vi "Behaviors and stuff in progress.vi"() -> ()   [LabVIEW 2016]
uses:
  <vilib>/platform/TimedLoop/XDataNode/XDataNode.xnode
  <vilib>/Platform/TimedLoop/XDataNode/nitl_modes.ctl
  <vilib>/Platform/TimedLoop/XDataNode/XDNodeRunTimeDep.lvlib
  <vilib>/Platform/TimedLoop/XDataNode/wakeup.ctl
  <vilib>/Platform/TimedLoop/XDataNode/timing_clust.ctl
  Intake Commands.ctl
  <vilib>/Rock Robotics/SystemInterfaces/DIO/FPGA_DIOPWMChannel.ctl
  <vilib>/Rock Robotics/WPI/PWM/WPI_PWMDeadband.ctl
  <vilib>/Rock Robotics/WPI/MotorControl/WPI_MotorControlType.ctl
  <vilib>/Rock Robotics/WPI/MotorControl/WPI_MotorControlDeviceRef.ctl
panel:
  in  "Softstop":dbl
  in  "bottomInvert":bool
  in  "topInvert":bool
  in  "RpmThreshold":dbl
  in  "RpmStableVal":dbl
  in  "?":T1
  in  "MotorControlDevRef 2":T2={"DeviceStatus"={"status"=FALSE, "code"=0, "source"=""}, "Type"=enum."PWM", "PWM"={"PWM Channel"=enum."Invalid", "DeadBand"={"Name"="", "maxPositivePwm"=0, "minPositivePwm"=0, "centerPwm"=0, "maxNegativePwm"=0, "minNegativePwm"=0, "angularRange"=0}}, "CAN"={"Device Number"=0, "SetOutput VI Ref"=variant(enum8{"Percent VBus", "Current", "Speed", "Position", "Voltage"} enum."Percent VBus"), "GetOutput VI Ref"=variant(refnum<k1> refnum), "Enable VI Ref"=variant(dbl 12.0), "Disable VI Ref"=variant(enum8{"Percent VBus", "Speed", "Position", "Slave", "Unchanged / Invalid"} enum."Percent VBus"), "Data"=variant}, "Invert"=FALSE}
  in  "Carousel Invert?":bool
  in  "Conveyor Invert?":bool
  in  "bottomPIDF":T6
  in  "topPIDF":T7
  in  "Desired Angle 2":dbl
  in  "Desired Angle":dbl
  in  "Carousel motorInput":dbl
  in  "Conveyor motorInput":dbl
  in  "output range":cluster{"output high":dbl, "output low":dbl}={"output high"=1.0, "output low"=-1.0}
  in  "PID gains":T8={"proportional gain (Kc)"=1.0, "integral time (Ti, min)"=0.01, "derivative time (Td, min)"=0.0} {"derivative time (Td, min)" format="%.3f"; "integral time (Ti, min)" format="%.3f"; "proportional gain (Kc)" format="%.3f"}
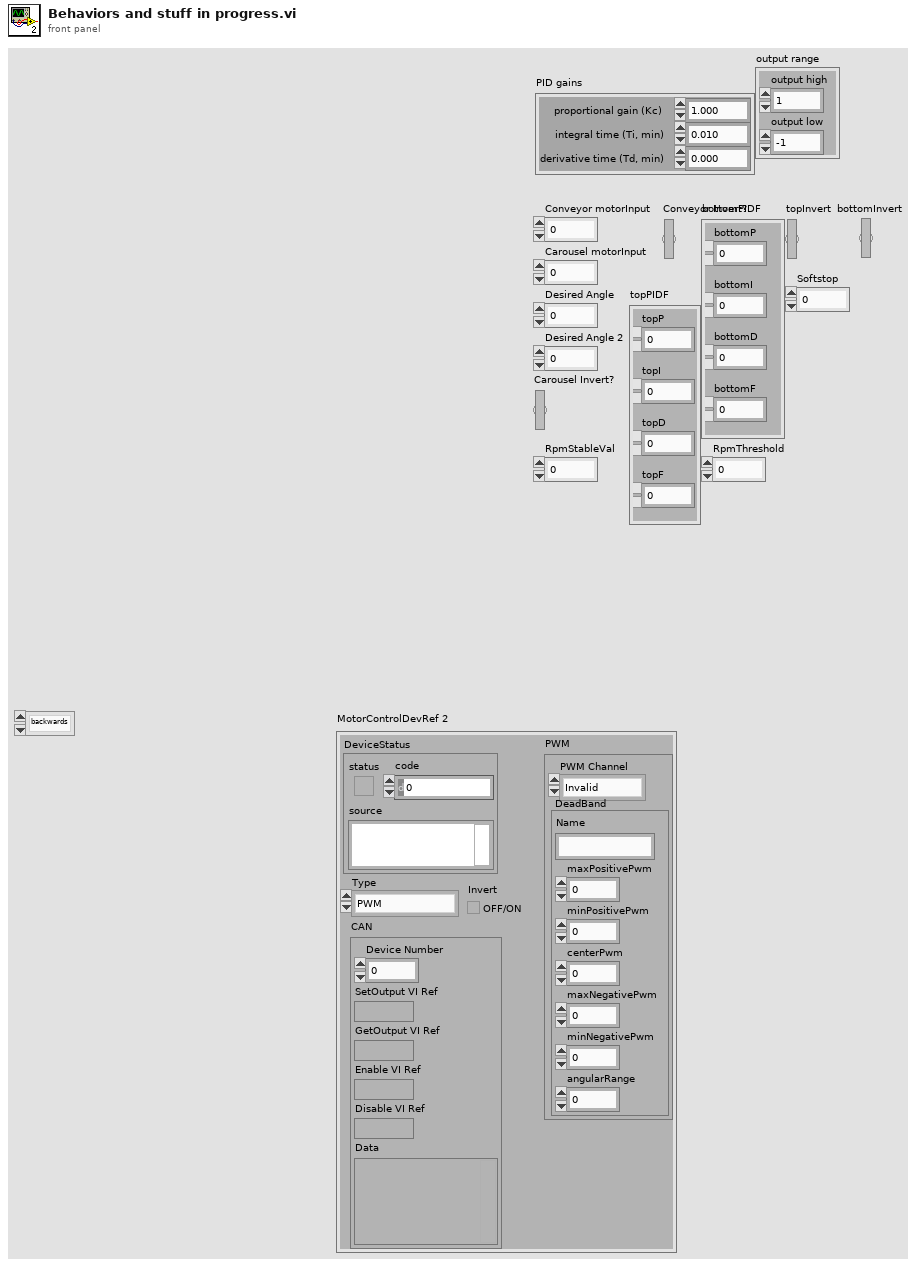
[diagram p1: front panel]
types:
  T1 = typedef "Intake Commands.ctl" = enum16{"backwards", "stop", "forward"}
  T2 = typedef "WPI_MotorControlDeviceRef.ctl" = cluster{"DeviceStatus":errorcluster, "Type":T3, "PWM":cluster{"PWM Channel":T4, "DeadBand":T5}, "CAN":cluster{"Device Number":u8, "SetOutput VI Ref":variant, "GetOutput VI Ref":variant, "Enable VI Ref":variant, "Disable VI Ref":variant, "Data":variant}, "Invert":bool}
  T3 = typedef "WPI_MotorControlType.ctl" = enum16{"PWM", "CAN"}
  T4 = typedef "FPGA_DIOPWMChannel.ctl" = enum8{"PWM 0", "PWM 1", "PWM 2", "PWM 3", "PWM 4", "PWM 5", "PWM 6", "PWM 7", "PWM 8", "PWM 9", "PWM MXP 0", "PWM MXP 1", "PWM MXP 2", "PWM MXP 3", "PWM MXP 4", "PWM MXP 5", "PWM MXP 6", "PWM MXP 7", "PWM MXP 8", "PWM MXP 9", "Invalid"}
  T5 = typedef "WPI_PWMDeadband.ctl" = cluster{"Name":string, "maxPositivePwm":i32, "minPositivePwm":i32, "centerPwm":i32, "maxNegativePwm":i32, "minNegativePwm":i32, "angularRange":u16}
  T6 = cluster{"bottomP":dbl, "bottomI":dbl, "bottomD":dbl, "bottomF":dbl}
  T7 = cluster{"topP":dbl, "topI":dbl, "topD":dbl, "topF":dbl}
  T8 = cluster{"proportional gain (Kc)":dbl, "integral time (Ti, min)":dbl, "derivative time (Td, min)":dbl}
  T9 = typedef "WPI_DigitalInputDevRef.ctl" = cluster{"DevStatus":errorcluster, "DIO Channel":T10}
  T10 = typedef "FPGA_DIOChannel.ctl" = enum8{"DIO 0", "DIO 1", "DIO 2", "DIO 3", "DIO 4", "DIO 5", "DIO 6", "DIO 7", "DIO 8", "DIO 9", "DIO MXP 0", "DIO MXP 1", "DIO MXP 2", "DIO MXP 3", "DIO MXP 4", "DIO MXP 5", "DIO MXP 6", "DIO MXP 7", "DIO MXP 8", "DIO MXP 9", "DIO MXP 10", "DIO MXP 11", "DIO MXP 12", "DIO MXP 13", "DIO MXP 14", "DIO MXP 15", "SPI Port CS1", "SPI Port CS2", "SPI Port CS3", "SPI Port MISO", "SPI Port MOSI", "Invalid"}
  T11 = typedef "XDNodeRunTimeDep.lvlib/timing_clust.ctl" = cluster{"Expected End [f-1]":u64, "Actual End [f-1]":u64, "Finished Late? [f-1]":bool, "Expected End [i-1]":u64, "Actual End [i-1]":u64, "Finished Late? [i-1]":bool, "Expected Start [i]":u64, "Actual Start [i]":u64, "Expected Start [f]":u64, "Actual Start [f]":u64, "Source Name":string, "Structure Name":string, "Period":i64, "Deadline":i64, "Offset":i64, "Start":i64, "Priority":i32, "Timeout":i32, "Mode":T12, "Wakeup Reason":T13, "Error":errorcluster, "Source Type":string, "Secondary Source Type":string, "Global End Time":u64, "Global Start Time":u64, "Frame Duration":u64, "Iteration Duration":u64, "Assigned CPU":i32, "I/O Scan Engine Mode":u32}
  T12 = typedef "XDNodeRunTimeDep.lvlib/nitl_modes.ctl" = enum32{"No Change", "Process missed periods, maintain original phase", "Discard missed periods, maintain original phase", "Process missed periods, ignore original phase", "Discard missed periods, ignore original phase"}
  T13 = typedef "XDNodeRunTimeDep.lvlib/wakeup.ctl" = enum32{"Normal", "Aborted", "Asynchronous wakeup", "Timing source error", "Timed loop error", "Timeout"}
  T14 = typedef "WPI_CANTalonSRX_GlobalStatus.ctl" = cluster{"Applied Throttle":dbl, "Module Enabled":bool, "CAN Error":errorcluster, "Closed Loop Error":dbl, "Forward Limit Switch Closed":bool, "Reverse Limit Switch Closed":bool, "Sensor Position":dbl, "Sensor Velocity":dbl, "Current":dbl, "Sticky Fault - Over Temp":bool, "Sticky Fault - Under Voltage":bool, "Sticky Fault - Forward Limit":bool, "Sticky Fault - Reverse Limit":bool, "Sticky Fault - Forward Soft Limit":bool, "Sticky Fault - Reverse Soft Limit":bool, "Brake is Enabled":bool, "Encoder Position":dbl, "Encoder Velocity":dbl, "Encoder Index Count":dbl, "Encoder A Pin State":bool, "Encoder B Pin State":bool, "Encoder Index Pin State":bool, "Analog In":dbl, "Analog In Velocity":dbl, "Temperature (C)":dbl, "Battery Voltage":dbl, "Control 5 Is Supported":bool, "Current Profile Slot Select":dbl, "Pos Div 8":bool, "Vel Div 4":bool, "Pulse Width Position":i32, "Pulse Width Velocity":i32, "Pulse Width Rise To Rise (us)":i32, "Pulse Width Rise To Fall (us)":i32, "Mot Prof Active Is Under Run":bool, "Mot Prof Active Has Under Run":bool, "Mot Prof Active Is Last":bool, "Mot Prof Active Velocity Only":bool, "Mot Prof Active Is Valid":bool, "Mot Prof Buffer Is Full":bool, "Mot Prof Active Profile Slot Select":i32, "Mot Prof NextID":i32, "Mot Prof Count":i32, "Mot Prof Active Velocity":dbl, "Mot Prof Active Position":dbl, "Mot Prof Output Enable":i32}
  T15 = cluster{"Encoder Velocity":dbl, "Desired Angle":dbl}
  T16 = cluster{"Desired Angle 2":dbl, "Encoder Velocity":dbl}
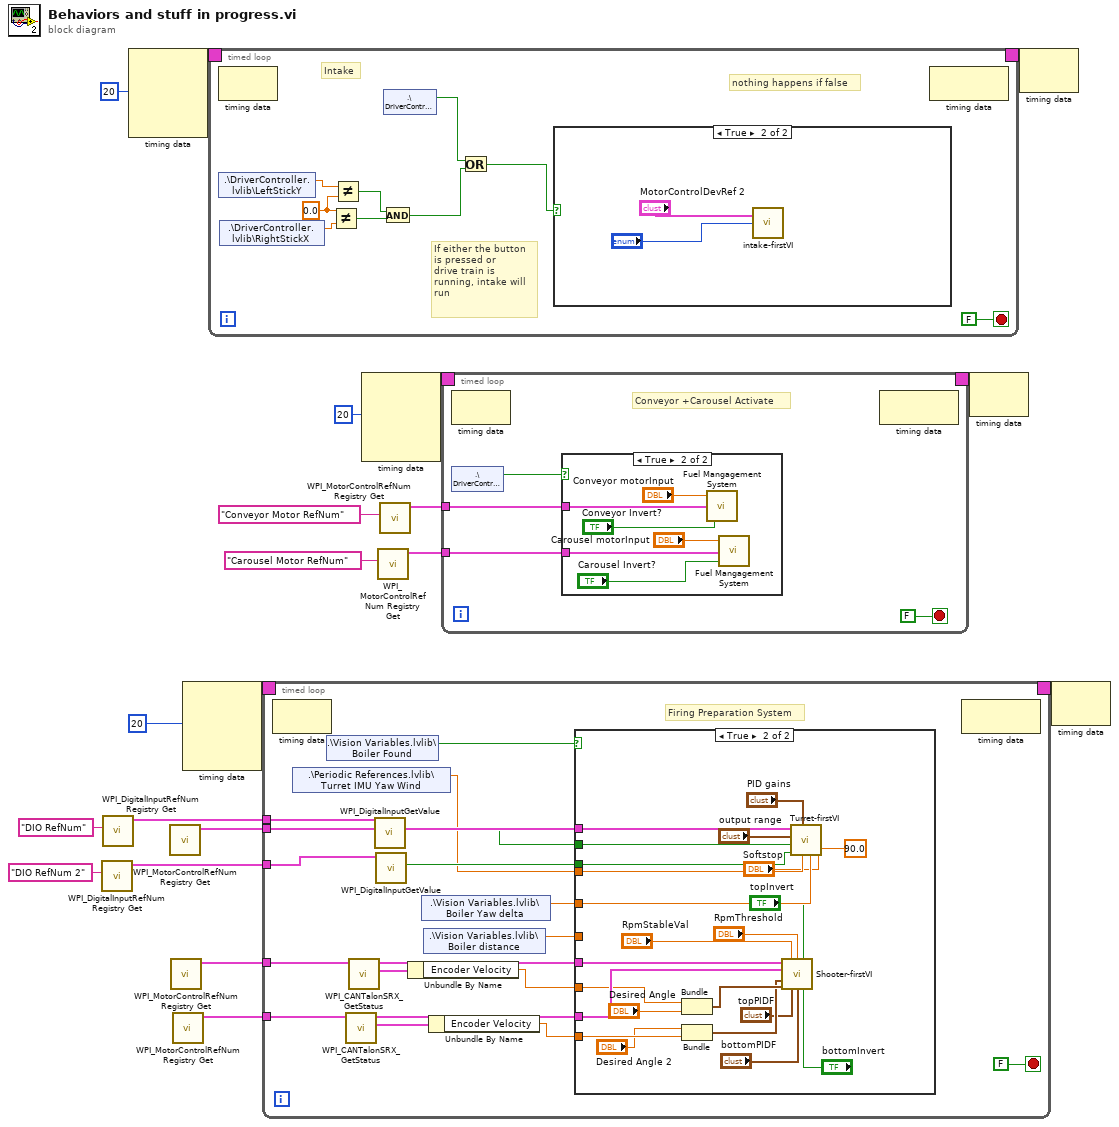
[diagram p0: block diagram]
diagram:
  n1 = call <vilib>:"WPI_DigitalInputRefNum Registry Get.vi"("refnum name"="DIO RefNum 2") -> ("DigitalInputDevRef"=w10:T9)  [unwired: 9 in, 1 out]
  n2 = call <vilib>:"WPI_DigitalInputRefNum Registry Get.vi"("refnum name"="DIO RefNum") -> ("DigitalInputDevRef"=w11:T9)  [unwired: 9 in, 1 out]
  n3 = node-c288(i64 20 ("Period")) -> (w3:T11)  [unwired: 3 in]
  n4 = call <vilib>:"WPI_MotorControlRefNum Registry Get.vi"() -> ("MotorControlDevRef"=w20:T2)  [unwired: 10 in, 1 out]
  n5 = call <vilib>:"WPI_MotorControlRefNum Registry Get.vi"() -> ("MotorControlDevRef"=w18:T2)  [unwired: 10 in, 1 out]
  n6 = call <vilib>:"WPI_MotorControlRefNum Registry Get.vi"() -> ("MotorControlDevRef"=w19:T2)  [unwired: 10 in, 1 out]
  n7 = node-c288(i64 20 ("Period")) -> (w17:T11)  [unwired: 3 in]
  n8 = timed-loop {
    timing: w3 -> [_]
    timing-out: [_] -> w2
    stop <- FALSE stop-if-true
    w22 = 0.0 ("x")
    # "Intake"
    # "If either the button \nis pressed or \ndrive train is\nrunning, intake will\nrun"
    # "nothing happens if false"
    n9 = node-c288() -> ()  [unwired: 1 in, 1 out]
    n10 = shared-variable ".\\DriverController.lvlib\\LeftStickY"() -> (w24:dbl)  [unwired: 1 in, 1 out]
    n11 = shared-variable ".\\DriverController.lvlib\\RightStickX"() -> (w23:dbl)  [unwired: 1 in, 1 out]
    n12 = Not Equal?(x=w22, y=w23) -> (x != y?=w26:bool)
    n13 = Not Equal?(x=w24, y=w22) -> (x != y?=w25:bool)
    n14 = And(x=w25, y=w26) -> (x .and. y?=w21:bool)
    n15 = shared-variable ".\\DriverController.lvlib\\A"() -> (w27:bool)  [unwired: 1 in, 1 out]
    n16 = Or(x=w27, y=w21) -> (x .or. y?=w29:bool)
    n17 = case shown="True" w29 {
      frame False {
      }
      frame True {
        n18 = call "intake-firstVI.vi"(0:"?", "MotorControlDevRef"="MotorControlDevRef 2") -> ()
      }
    }
    n19 = node-c288() -> ()  [unwired: 1 in, 1 out]
  }
  n20 = timed-loop {
    tunnel: w20 -> [w49]
    tunnel: w19 -> [w41]
    tunnel: w18 -> [w44]
    timing: w17 -> [_]
    timing-out: [_] -> w16
    tunnel: w11 -> [w47]
    tunnel: w10 -> [w48]
    stop <- FALSE stop-if-true
    # "Firing Preparation System"
    n21 = node-c288() -> ()  [unwired: 1 in, 1 out]
    n22 = shared-variable ".\\Periodic References.lvlib\\Turret IMU Yaw Wind"() -> (w38:dbl)  [unwired: 1 in, 1 out]
    n23 = shared-variable ".\\Vision Variables.lvlib\\Boiler Found"() -> (w51:bool)  [unwired: 1 in, 1 out]
    n24 = call <vilib>:"WPI_CANTalonSRX_GetStatus.vi"("CAN Talon SRX Ref"=w41) -> ("Talon SRX Status"=w39:T14, "CAN Talon SRX Ref"=w40:T2)  [unwired: 8 in, 1 out]
    n25 = call <vilib>:"WPI_CANTalonSRX_GetStatus.vi"("CAN Talon SRX Ref"=w44) -> ("Talon SRX Status"=w42:T14, "CAN Talon SRX Ref"=w43:T2)  [unwired: 8 in, 1 out]
    n26 = call <vilib>:"WPI_DigitalInputGetValue.vi"("DigitalInputDevRef"=w47) -> ("Value"=w46:bool)  [unwired: 8 in, 2 out]
    n27 = call <vilib>:"WPI_DigitalInputGetValue.vi"("DigitalInputDevRef"=w48) -> ("Value"=w45:bool)  [unwired: 8 in, 2 out]
    n28 = Unbundle By Name(w42) -> ("Encoder Velocity"=w36:dbl)
    n29 = shared-variable ".\\Vision Variables.lvlib\\Boiler Yaw delta"() -> (w37:dbl)  [unwired: 1 in, 1 out]
    n30 = shared-variable ".\\Vision Variables.lvlib\\Boiler distance"() -> (w34:dbl)  [unwired: 1 in, 1 out]
    n31 = Unbundle By Name(w39) -> ("Encoder Velocity"=w35:dbl)
    n32 = case shown="True" w51 {
      tunnel: w49 -> [_ w76]
      tunnel: w40 -> [_ w75]
      tunnel: w43 -> [_ w74]
      tunnel: w46 -> [_ w71]
      tunnel: w45 -> [_ w70]
      tunnel: w38 -> [_ w69]
      tunnel: w37 -> [_ w68]
      tunnel: w36 -> [_ w67]
      tunnel: w35 -> [_ w64]
      tunnel: w34 -> [_ _]
      frame False {
      }
      frame True {
        n33 = Bundle("Encoder Velocity"=w67, "Desired Angle"="Desired Angle") -> (w65:T15)  [unwired: 1 in]
        n34 = Bundle("Desired Angle 2"="Desired Angle 2", "Encoder Velocity"=w64) -> (w62:T16)  [unwired: 1 in]
        n35 = call "Shooter-firstVI.vi"("bottomWheelMotor"=w74, "RpmStableVal"="RpmStableVal", "RpmThreshold"="RpmThreshold", "topInvert"="topInvert", "topWheelMotor"=w75, "topWheel"=w62, "bottomWheel"=w65, "topPIDF"="topPIDF", "bottomPIDF"="bottomPIDF", "bottomInvert"="bottomInvert") -> ()  [unwired: 5 in, 1 out]
        n36 = call "Turret-firstVI.vi"("Softstop"="Softstop", "shooter range"=90.0, "desired Angle"=w68, "Current angle"=w69, "PID gains"="PID gains", "Negative soft stop"=w70, "Positive soft stop"=w71, "output range"="output range", "MotorControlDevRef"=w76) -> ()  [unwired: 2 in, 1 out]
      }
    }
    n37 = node-c288() -> ()  [unwired: 1 in, 1 out]
  }
  n38 = node-c288(i64 20 ("Period")) -> (w15:T11)  [unwired: 3 in]
  n39 = call <vilib>:"WPI_MotorControlRefNum Registry Get.vi"("refnum name"="Carousel Motor RefNum") -> ("MotorControlDevRef"=w7:T2)  [unwired: 9 in, 1 out]
  n40 = call <vilib>:"WPI_MotorControlRefNum Registry Get.vi"("refnum name"="Conveyor Motor RefNum") -> ("MotorControlDevRef"=w6:T2)  [unwired: 9 in, 1 out]
  n41 = timed-loop {
    timing: w15 -> [_]
    timing-out: [_] -> w14
    tunnel: w7 -> [w78]
    tunnel: w6 -> [w77]
    stop <- FALSE stop-if-true
    # "Conveyor +Carousel Activate"
    n42 = node-c288() -> ()  [unwired: 1 in, 1 out]
    n43 = shared-variable ".\\DriverController.lvlib\\Y"() -> (w79:bool)  [unwired: 1 in, 1 out]
    n44 = case shown="True" w79 {
      tunnel: w78 -> [_ w88]
      tunnel: w77 -> [_ w87]
      frame False {
      }
      frame True {
        n45 = call "Fuel Mangagement System.vi"("Invert?"="Conveyor Invert?", "hopperDevRef"=w87, "motorInput"="Conveyor motorInput") -> ()  [unwired: 1 out]
        n46 = call "Fuel Mangagement System.vi"("Invert?"="Carousel Invert?", "hopperDevRef"=w88, "motorInput"="Carousel motorInput") -> ()  [unwired: 1 out]
      }
    }
    n47 = node-c288() -> ()  [unwired: 1 in, 1 out]
  }
  n48 = node-c288(w14) -> ()  [unwired: 1 out]
  n49 = node-c288(w2) -> ()  [unwired: 1 out]
  n50 = node-c288(w16) -> ()  [unwired: 1 out]
